vi "AB_Engine_Should_Assume_Refee_Links.vi"(10 "Refee":T2, 11 "Refer":T2) -> (3 "Assume refee links?":bool)   [LabVIEW 2020]
uses:
  <vilib>/Utility/lvfile.llb/LVFileType.ctl
  <vilib>/Utility/lvfile.llb/NI_FileType.lvlib
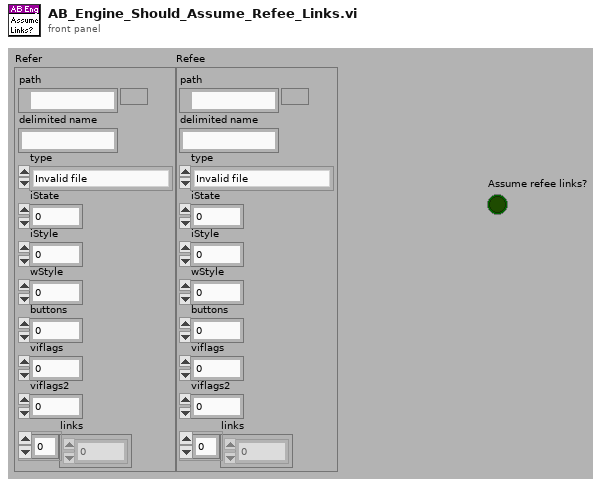
[diagram p1: front panel]
types:
  T1 = typedef "NI_FileType.lvlib/LVFileType.ctl" = enum32{"Invalid file", "Unknown type", "Instrument", "Control", "Polymorphic VI", "Project", "Library", "LVClass", "XControl", "XNode", "Shared library", ".NET assembly", "ActiveX interface", "CIN", "Run-time menu", "Palette menu", "Help file", "LLB", "XNode Edit Dependency", "Class Private Data Control", "Statechart", "MathScript .m file", "Ladder Diagram", "LVLibp", "XNode Build Dependency"}
  T2 = cluster{"path":path, "delimited name":string, "type":T1, "iState":u32, "iStyle":u16, "wStyle":u16, "buttons":u16, "viflags":u32, "viflags2":u32, "links":u32[]}
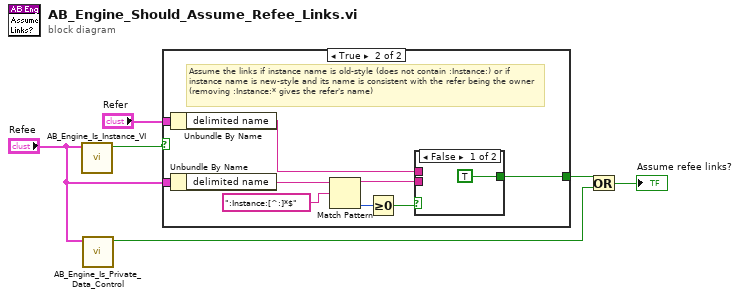
[diagram p0: block diagram]
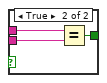
[diagram p3: hidden frame]
diagram:
  n1 = call <vilib>:"AB_Engine_Is_Instance_VI.vi"("File"="Refee") -> ("Is Instance VI?"=w6:bool)  [unwired: 10 out]
  n2 = call <vilib>:"AB_Engine_Is_Private_Data_Control.vi"("File"="Refee") -> ("Is Private Data Control?"=w2:bool)  [unwired: 10 out]
  n3 = case shown="True" w6 {
    selector: w6 -> [w7 _]
    tunnel: "Refee" -> [_ w16]
    tunnel: "Refer" -> [_ w15]
    tunnel: [w7 w12] -> w3
    frame False {
    }
    frame True {
      # "Assume the links if instance name is old-style (does not contain :Instance:) or if instance name is new-style and its name is consistent with the refer being the owner (removing :Instance:* gives the refer's name)"
      n4 = Unbundle By Name(w15) -> ("delimited name"=w14:string)
      n5 = Unbundle By Name(w16) -> ("delimited name"=w10:string)
      n6 = Match Pattern(string=w10, regular expression=":Instance:[^:]*$" ("search string/char (-)")) -> (before substring=w9:string, offset past match=w8:i32)  [unwired: 3 out]
      n7 = Greater Or Equal To 0?(x=w8) -> (x >= 0?=w13:bool)
      n8 = case shown="False" w13 {
        tunnel: w9 -> [_ w18]
        tunnel: w14 -> [_ w20]
        tunnel: [TRUE w19] -> w12
        frame False {
        }
        frame True {
          n9 = Equal?(x=w20, y=w18) -> (x = y?=w19:bool)
        }
      }
    }
  }
  n10 = Or(x=w3, y=w2) -> (x .or. y?=→"Assume refee links?":bool)
